vi "MSScript_Format_Wait.vi"(9 "ValueArray":string[](array[string]), 10 "TagArray":string[](array[string]), 11 "MSScript in":refnum<class "MSScript.lvclass">) -> (0 "ValueErrorArray":bool[](array[boolean]), 1 "TagErrorArray":bool[](array[boolean]), 2 "ParamErrorArray":bool[](array[boolean]), 3 "Data":variant, 4 "#ofParamError":bool)   [LabVIEW 2018, in "MSScript.lvclass"]
uses:
  MSScript.lvclass
  Ctl/MSEditorParam wait.ctl
  MSScript_Transform_Extended.vi
  MSScript_Transform_UInt.vi
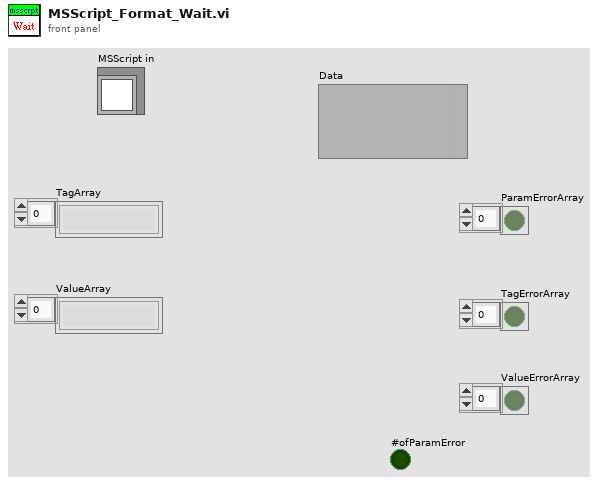
[diagram p1: front panel]
types:
  T1 = typedef "MSEditorParam wait.ctl" = cluster{"timeout":ext, "DI":u16, "edge":u16}
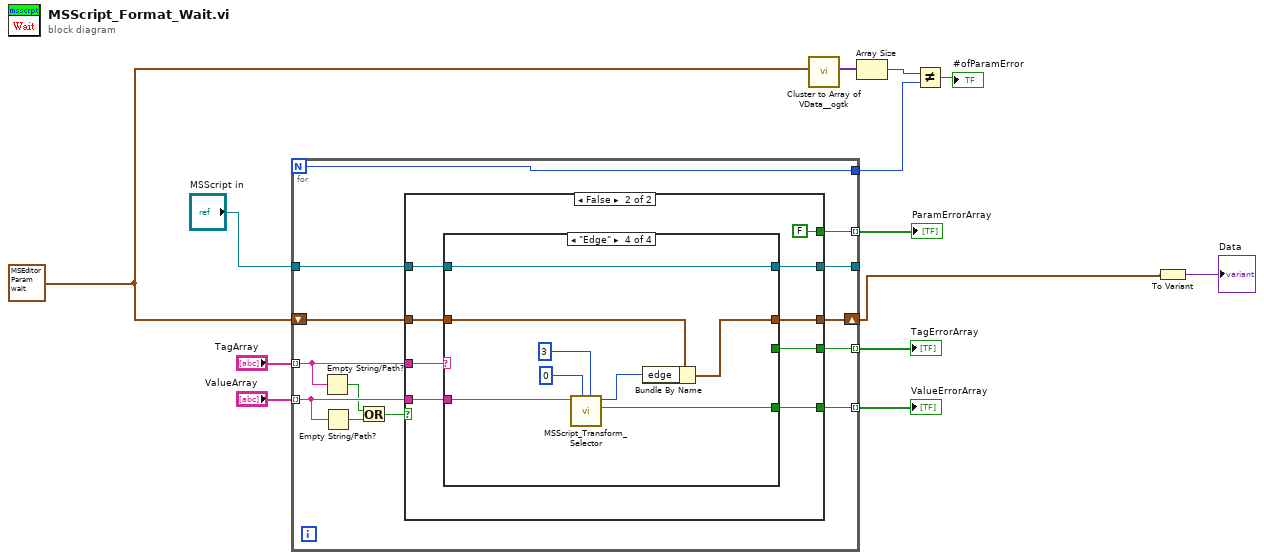
[diagram p0: block diagram]
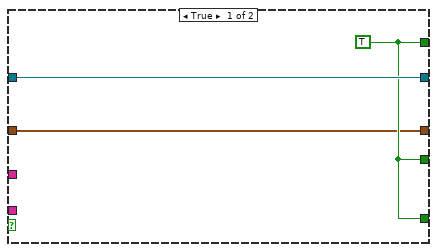
[diagram p2: hidden frame]
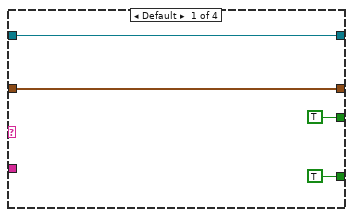
[diagram p3: hidden frame]
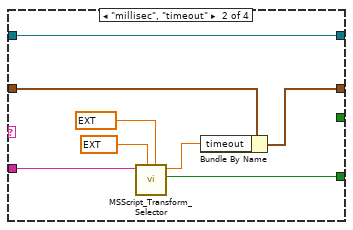
[diagram p4: hidden frame]
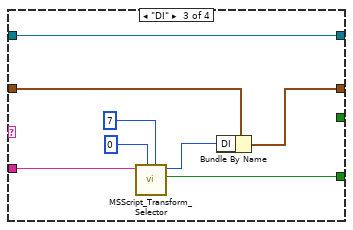
[diagram p5: hidden frame]
diagram:
  w4 = T1 {"timeout"=0.001, "DI"=0, "edge"=0} ("ParamValueType")
  n1 = for {
    N -> [w14]
    tunnel: "TagArray" -> [w22] mode=indexing
    tunnel: "ValueArray" -> [w21] mode=indexing
    tunnel: [w26] -> w11 mode=indexing
    tunnel: "MSScript in" -> [w25]
    tunnel: [w24] -> w10 mode=indexing
    tunnel: [w23] -> _
    tunnel: [w17] -> w9 mode=indexing
    shift-right: [w15] -> w2
    shift-left: w4 -> [w16]
    tunnel: [w14] -> w3
    n2 = Empty String/Path?(string/path=w22) -> (empty?=w19:bool)
    n3 = Empty String/Path?(string/path=w21) -> (empty?=w20:bool)
    n4 = Or(x=w19, y=w20) -> (x .or. y?=w18:bool)
    n5 = case shown="False" w18 {
      tunnel: [w28 w32] -> w26
      tunnel: w25 -> [w29 w36]
      tunnel: [w28 w33] -> w24
      tunnel: [w29 w30] -> w23
      tunnel: w22 -> [_ w35]
      tunnel: w21 -> [_ w34]
      tunnel: [w28 FALSE] -> w17
      tunnel: w16 -> [w27 w37]
      tunnel: [w27 w31] -> w15
      frame True {
        w28 = TRUE
      }
      frame False {
        n6 = case shown="\"Edge\"" w35 {
          tunnel: [TRUE _ _ _] -> w32
          tunnel: w36 -> [w40 w47 w55 w63]
          tunnel: w34 -> [_ w48 w56 w64]
          tunnel: [TRUE ("Value Error?") w50 w58 w66] -> w33
          tunnel: [w40 w47 w55 w63] -> w30
          tunnel: w37 -> [w39 w45 w53 w61]
          tunnel: [w39 w44 w52 w60] -> w31
          frame Default {
          }
          frame "millisec", "timeout" {
            n7 = call-poly "MSScript_Transform_Selector.vi"("upper limit (Inf)"=ext 60000.0 ("upper limit"), "lower limit (-Inf)"=ext 0.001 ("lower limit"), "Check_Str"=w48) -> ("Value Error?"=w50:bool, "Value Output"=w46:ext)  [unwired: 6 in, 1 out]
            n8 = Bundle By Name(cluster=w45, "timeout"=w46) -> (w44:T1)
          }
          frame "DI" {
            n9 = call-poly "MSScript_Transform_Selector.vi"("upper limit"=u64 7, "lower limit"=u64 0, "string in"=w56) -> ("Value Error?"=w58:bool, "Value Output"=w54:u64)  [unwired: 6 in, 1 out]
            n10 = Bundle By Name(cluster=w53, "DI"=w54) -> (w52:T1)
          }
          frame "Edge" {
            n11 = call-poly "MSScript_Transform_Selector.vi"("upper limit"=u64 3, "lower limit"=u64 0, "string in"=w64) -> ("Value Error?"=w66:bool, "Value Output"=w62:u64)  [unwired: 6 in, 1 out]
            n12 = Bundle By Name(cluster=w61, "edge"=w62) -> (w60:T1)
          }
        }
      }
    }
  }
  "TagErrorArray" <- w11
  "ValueErrorArray" <- w10
  "ParamErrorArray" <- w9
  n13 = call <userlib>:"Cluster to Array of VData__ogtk.vi"("Cluster"=w4) -> ("Array of VData"=w7:variant[])  [unwired: 9 in, 1 out]
  n14 = Array Size(array=w7) -> (size(s)=w6:i32)
  n15 = Not Equal?(x=w6, y=w3) -> (x != y?=→"#ofParamError":bool)
  n16 = To Variant(anything=w2) -> (Variant=→"Data":variant)
